vi "mupSetExpr.vi"(8 "error in (no error)":errorcluster, 10 "szExpr":string, 11 "muPar in":u64) -> (0 "error out":errorcluster, 3 "muPar out":u64)   [LabVIEW 2015, in "mupLib.lvlib"]
doc: "Set the expression string. Multiple expressions can be input using comma as delimiter."
uses:
  mupLib.lvlib
panel:
  # "Set the expression string. Multiple expressions can be input using comma as delimiter."
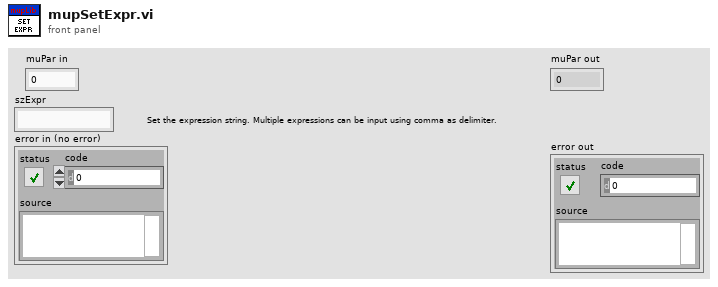
[diagram p1: front panel]
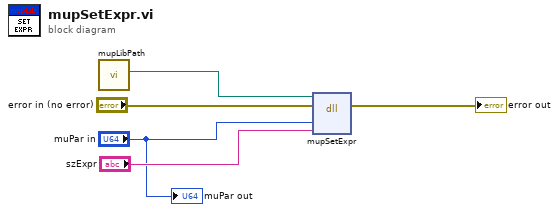
[diagram p0: block diagram]
diagram:
  n1 = call "mupLibPath.vi"() -> ("libmuparser path"=w1:path)  [unwired: 11 in]
  n2 = dll-call lib="usr/lib/x86_64-linux-gnu/libmuparser.so.2" fn="mupSetExpr"(path in=w1, error in="error in (no error)", "hParser"="muPar in", "szExpr"="szExpr") -> (error out=→"error out":errorcluster)  [unwired: 4 in, 1 out]
  "muPar out" <- "muPar in"
